vi "TestActuatorInterlock.vi"(3 "Input Value Boolean":bool, 4 "Input Value Double":dbl, 5 "Actuator_Name":string) -> (0 "Output Value Boolean":bool, 1 "Output Value Double":dbl, 2 "In Test Mode":bool)   [LabVIEW 2019]
doc: "This VI functions as an interlock, allowing operators to bypass the control logic for each actuator and test it using basic commands. This VI supports both floating point and boolean outputs. It requires integration with global variables storing the test signal and the operator's actuator selection. It is intended to integrate with the standard FRC 4265 control architecture."
panel:
  in  "Test actuator Name Selection [PLACEHOLDER]":string
  in  "Test Actuator Value [PLACEHOLDER]":dbl
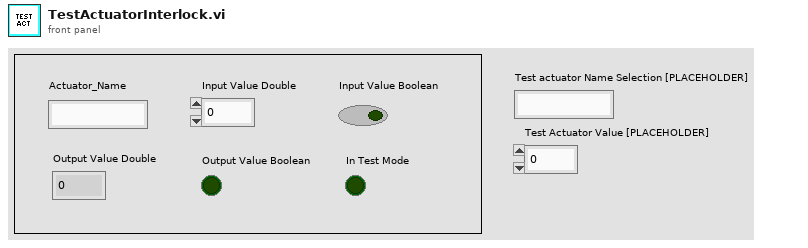
[diagram p1: front panel]
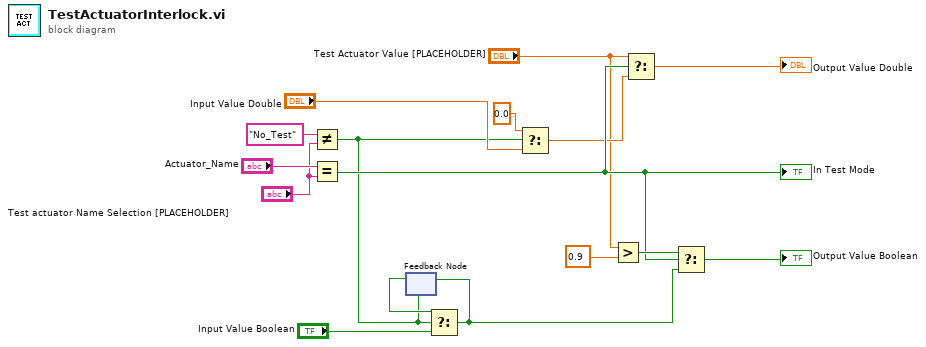
[diagram p0: block diagram]
diagram:
  n1 = Not Equal?(x="No_Test", y="Test actuator Name Selection [PLACEHOLDER]") -> (x != y?=w3:bool)
  n2 = Equal?(x="Actuator_Name", y="Test actuator Name Selection [PLACEHOLDER]") -> (x = y?=w12:bool)
  "In Test Mode" <- w12
  n3 = feedback #1(w3) -> (w4:bool)
  n4 = Select(t=w4, s=w3, f="Input Value Boolean") -> (s? t:f=w5:bool)
  n5 = feedback-in #1(w5) -> ()
  n6 = Select(t=0.0, s=w3, f="Input Value Double") -> (s? t:f=w7:dbl)
  n7 = Greater?(x="Test Actuator Value [PLACEHOLDER]", y=0.9) -> (0:w14:bool)
  n8 = Select(t="Test Actuator Value [PLACEHOLDER]", s=w12, f=w7) -> (s? t:f=→"Output Value Double":dbl)
  n9 = Select(t=w14, s=w12, f=w5) -> (s? t:f=→"Output Value Boolean":bool)
